vi "PTScanner.parameters 2 byteArray.vi"(1 "Parameters":T2(array[cluster]), 4 "nomValue":dbl) -> (15 "byteArray out":T1)   [LabVIEW 2014, in "PTScanner.lvlib"]
uses:
  PTScanner.lvlib
  CS_Core/CSSystem/CoreDefs/CoreDefs.rawDataType.ctl
  CS_Core/CSSystem/CoreLib/CoreLib.string 2 byte array.vi
  CS_Core/CSSystem/CoreLib/CoreLib.double 2 byte array.vi
  CS_Core/CSSystem/CoreLib/CoreLib.float 2 byte array.vi
  CS_Core/CSSystem/CoreLib/CoreLib.int 2 byte array.vi
  CS_Core/CSSystem/CoreLib/CoreLib.short 2 byte array.vi
  CS_Core/CSSystem/CoreLib/CoreLib.lvlib
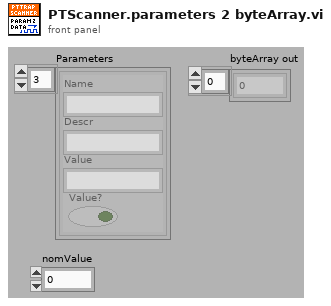
[diagram p1: front panel]
types:
  T1 = typedef "CoreDefs.rawDataType.ctl" = i8[]
  T2 = cluster{"Name":string, "Descr":string, "Value":string, "Value?":bool}[]
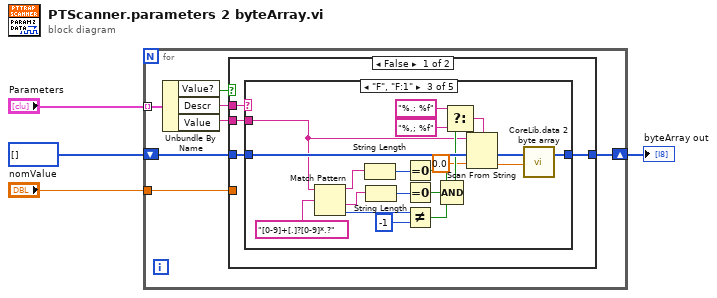
[diagram p0: block diagram]
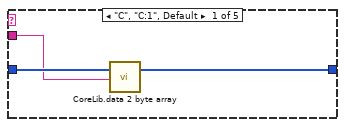
[diagram p2: hidden frame]
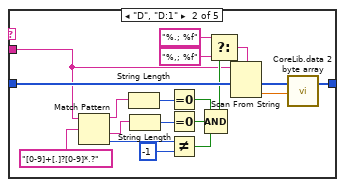
[diagram p3: hidden frame]
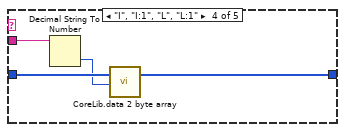
[diagram p4: hidden frame]
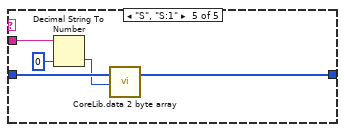
[diagram p5: hidden frame]
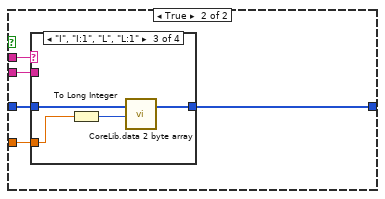
[diagram p6: hidden frame]
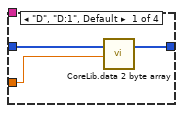
[diagram p7: hidden frame]
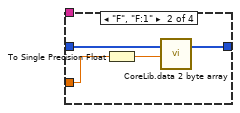
[diagram p8: hidden frame]
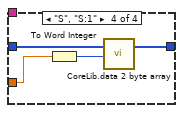
[diagram p9: hidden frame]
diagram:
  n1 = for {
    tunnel: "Parameters" -> [w11] mode=indexing
    shift-right: [w7] -> w1
    shift-left: T1 [] ("Data") -> [w6]
    tunnel: "nomValue" -> [w5]
    n2 = Unbundle By Name(w11) -> ("Value?"=w10:bool, "Descr"=w9:string, "Value"=w8:string)
    n3 = case shown="False" w10 {
      tunnel: w9 -> [w15 w69]
      tunnel: w8 -> [w14 w68]
      tunnel: [w13 w67] -> w7
      tunnel: w6 -> [w12 w66]
      tunnel: w5 -> [_ w65]
      frame False {
        n4 = case shown="\"F\", \"F:1\"" w15 {
          tunnel: w14 -> [w16 w20 w39 w57 w61]
          tunnel: [w18 w36 w55 w59 w64] -> w13
          tunnel: w12 -> [w17 w35 w54 w58 w63]
          frame "C", "C:1", Default {
            n5 = call-poly "CoreLib.data 2 byte array.vi"("byteArray"=w17, "string"=w16) -> ("byteArray out"=w18:T1)  [unwired: 17 in]
          }
          frame "D", "D:1" {
            n6 = Match Pattern(string=w20, regular expression="[0-9]+[.]?[0-9]*.?") -> (before substring=w27:string, after substring=w28:string, offset past match=w26:i32)  [unwired: 1 in, 1 out]
            n7 = String Length(string=w27) -> (length=w29:i32)
            n8 = String Length(string=w28) -> (length=w30:i32)
            n9 = Equal To 0?(x=w29) -> (x = 0?=w32:bool)
            n10 = Equal To 0?(x=w30) -> (x = 0?=w33:bool)
            n11 = Not Equal?(x=w26, y=-1) -> (x != y?=w34:bool)
            n12 = Compound Arithmetic op=AND(w32, w33, w34) -> (w21:bool)
            n13 = Select(t="%.; %f" ("format string"), s=w21, f="%,; %f" ("format string")) -> (s? t:f=w22:string)
            n14 = Scan From String(format string=w22, input string=w20) -> (output 1=w19:dbl)  [unwired: 3 in, 3 out]
            n15 = call-poly "CoreLib.data 2 byte array.vi"("byteArray"=w35, "f64"=w19) -> ("byteArray out"=w36:T1)  [unwired: 17 in]
          }
          frame "F", "F:1" {
            n16 = Match Pattern(string=w39, regular expression="[0-9]+[.]?[0-9]*.?") -> (before substring=w46:string, after substring=w47:string, offset past match=w45:i32)  [unwired: 1 in, 1 out]
            n17 = String Length(string=w46) -> (length=w48:i32)
            n18 = String Length(string=w47) -> (length=w49:i32)
            n19 = Equal To 0?(x=w48) -> (x = 0?=w51:bool)
            n20 = Equal To 0?(x=w49) -> (x = 0?=w52:bool)
            n21 = Not Equal?(x=w45, y=-1) -> (x != y?=w53:bool)
            n22 = Compound Arithmetic op=AND(w51, w52, w53) -> (w40:bool)
            n23 = Select(t="%.; %f" ("format string"), s=w40, f="%,; %f" ("format string")) -> (s? t:f=w41:string)
            n24 = Scan From String(format string=w41, input string=w39, default 1=sgl 0.0) -> (output 1=w37:sgl)  [unwired: 2 in, 3 out]
            n25 = call-poly "CoreLib.data 2 byte array.vi"("byteArray"=w54, "f32"=w37) -> ("byteArray out"=w55:T1)  [unwired: 17 in]
          }
          frame "I", "I:1", "L", "L:1" {
            n26 = Decimal String To Number(string=w57) -> (number=w56:i32)  [unwired: 2 in, 1 out]
            n27 = call-poly "CoreLib.data 2 byte array.vi"("byteArray"=w58, "i32"=w56) -> ("byteArray out"=w59:T1)  [unwired: 17 in]
          }
          frame "S", "S:1" {
            n28 = Decimal String To Number(string=w61, default (0L)=i16 0) -> (number=w60:i16)  [unwired: 1 in, 1 out]
            n29 = call-poly "CoreLib.data 2 byte array.vi"("byteArray"=w63, "i16"=w60) -> ("byteArray out"=w64:T1)  [unwired: 17 in]
          }
        }
      }
      frame True {
        n30 = case shown="\"I\", \"I:1\", \"L\", \"L:1\"" w69 {
          tunnel: w68 -> [_ _ _ _]
          tunnel: [w72 w76 w80 w84] -> w67
          tunnel: w66 -> [w71 w75 w79 w83]
          tunnel: w65 -> [w70 w74 w78 w82]
          frame "D", "D:1", Default {
            n31 = call-poly "CoreLib.data 2 byte array.vi"("byteArray"=w71, "f64"=w70) -> ("byteArray out"=w72:T1)  [unwired: 17 in]
          }
          frame "F", "F:1" {
            n32 = To Single Precision Float(number=w74) -> (single precision float=w73:sgl)
            n33 = call-poly "CoreLib.data 2 byte array.vi"("byteArray"=w75, "f32"=w73) -> ("byteArray out"=w76:T1)  [unwired: 17 in]
          }
          frame "I", "I:1", "L", "L:1" {
            n34 = To Long Integer(number=w78) -> (32bit integer=w77:i32)
            n35 = call-poly "CoreLib.data 2 byte array.vi"("byteArray"=w79, "i32"=w77) -> ("byteArray out"=w80:T1)  [unwired: 17 in]
          }
          frame "S", "S:1" {
            n36 = To Word Integer(number=w82) -> (16bit integer=w81:i16)
            n37 = call-poly "CoreLib.data 2 byte array.vi"("byteArray"=w83, "i16"=w81) -> ("byteArray out"=w84:T1)  [unwired: 17 in]
          }
        }
      }
    }
  }
  "byteArray out" <- w1
